vi "Get_DSC_Vals.vi"(8 "Machine":string, 9 "Shared Variable Control":refnum<k21>, 10 "Name":string, 11 "Authorization Header":T1[](array[typedef])) -> ()   [LabVIEW 2016]
uses:
  <vilib>/addons/_JKI.lib/REST Client/classes/REST Client/HTTP Header.ctl
  <vilib>/LVH/i3 JSON/JSON Parsing/Get Object Parameter Files/Get Object Parameter - Object.vi
  <vilib>/LVH/i3 JSON/JSON Parsing/Get Object Parameter Files/Get Object Parameter - String.vi
  <vilib>/addons/_JKI.lib/REST Client/classes/REST Client/REST Client.lvclass
  <vilib>/addons/_JKI.lib/Serialization/JSON/JKI JSON Serialization.lvlib
  <vilib>/LVH/i3 JSON/i3-json.lvlib
panel:
  in  "OK":bool
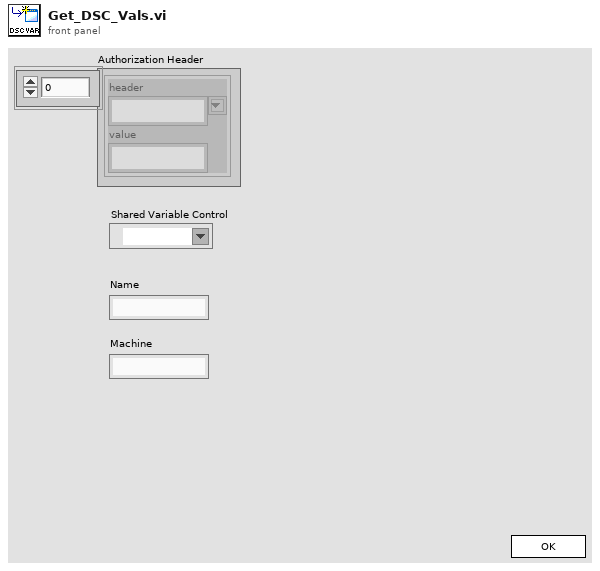
[diagram p1: front panel]
types:
  T1 = typedef "REST Client.lvlib/REST Client.lvclass/HTTP Header.ctl" = cluster{"header":string, "value":string}
  T2 = enum32{"Invalid", "Standard", "Closed", "Hidden", "Minimized", "Maximized"}
  T3 = enum32{"invalid app kind", "Development System", "Run Time System", "Student Edition", "Embedded LabVIEW", "Evaluation", "Custom"}
  T4 = cluster{"Core":cluster{"Current VI Reference":refnum<vi>, "Close Panel on Exit?":bool}, "New Reference":string, "Array of DSC References":cluster{string, string}[], "Authorization Header":T1[], "GID":string, "Name":string, "trimmed string":string, "Section GID":string}
  T5 = cluster{"Current VI Reference":refnum<vi>, "Close Panel on Exit?":bool}
  T6 = cluster{"data":cluster{"id":i32, "gid":string, "name":string, "resource_type":string}[]}
  T7 = cluster{"id":i32, "gid":string, "name":string, "resource_type":string}[]
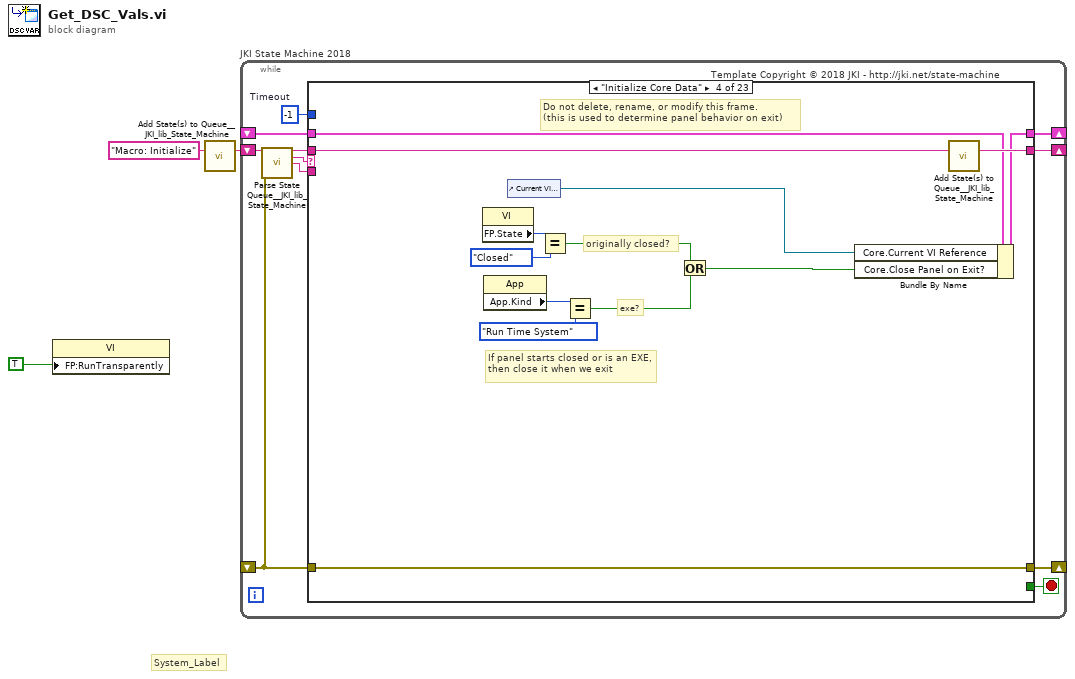
[diagram p0: block diagram]
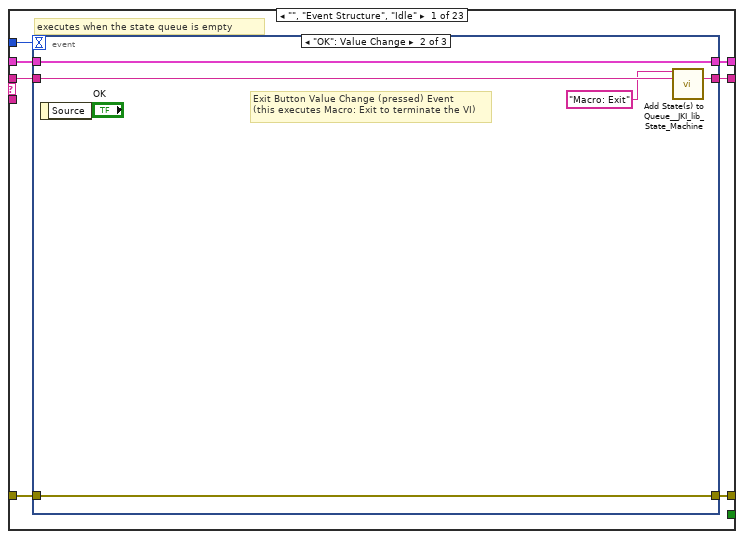
[diagram p2: hidden frame]
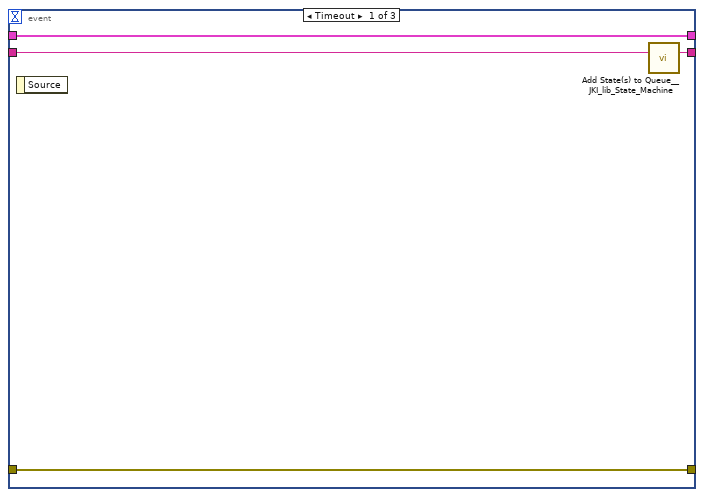
[diagram p3: hidden frame]
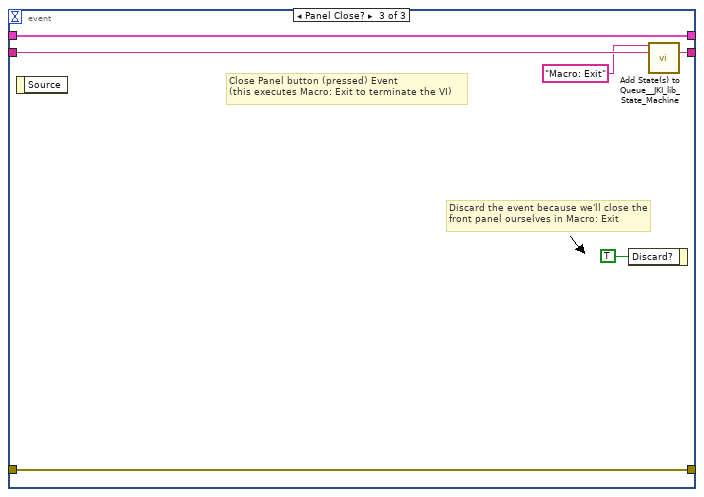
[diagram p4: hidden frame]
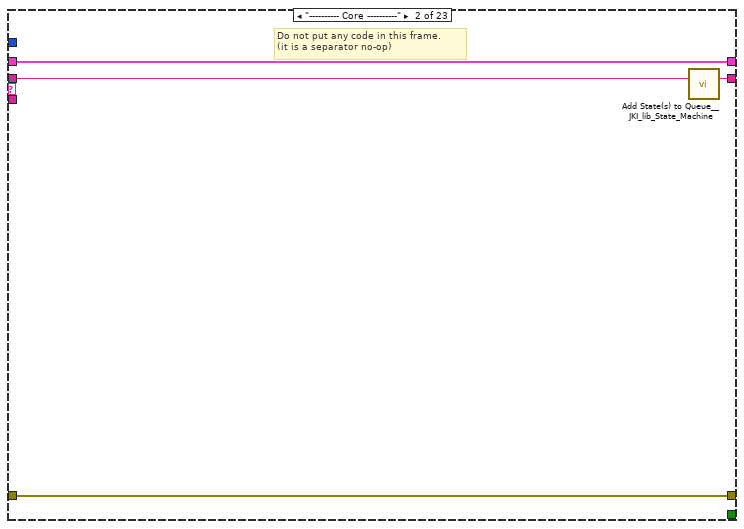
[diagram p5: hidden frame]
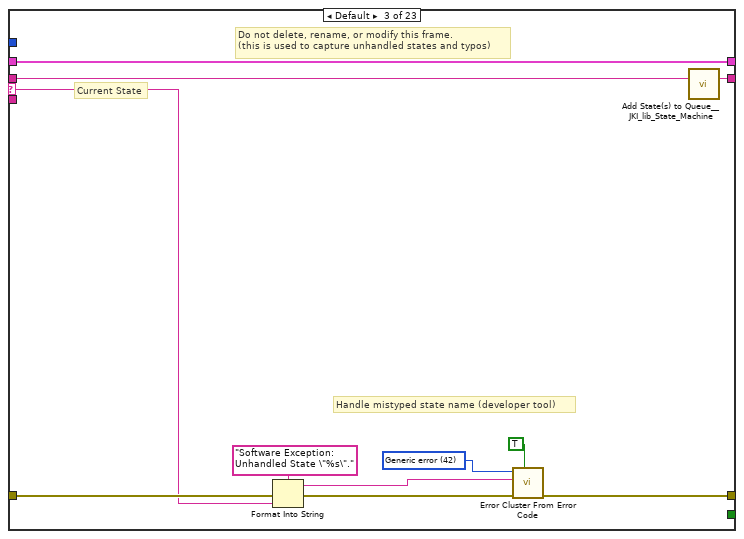
[diagram p6: hidden frame]
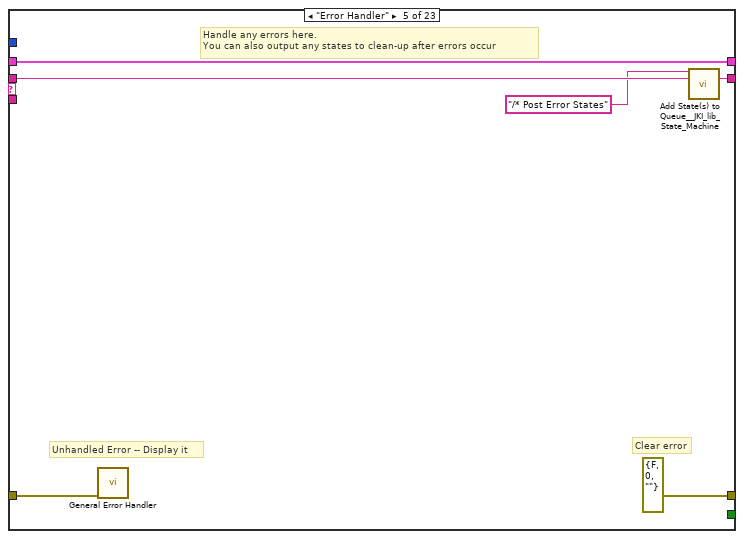
[diagram p7: hidden frame]
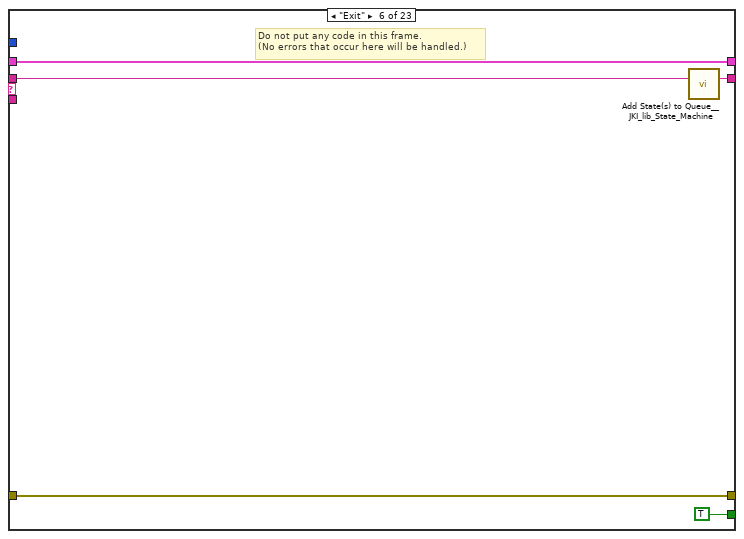
[diagram p8: hidden frame]
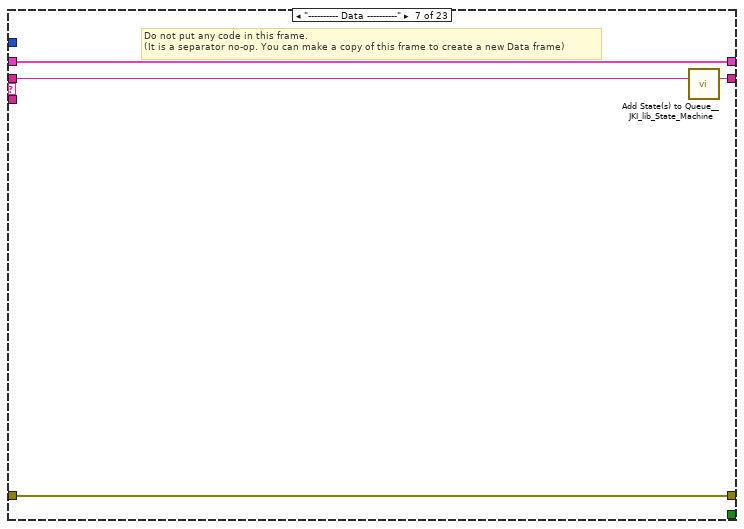
[diagram p9: hidden frame]
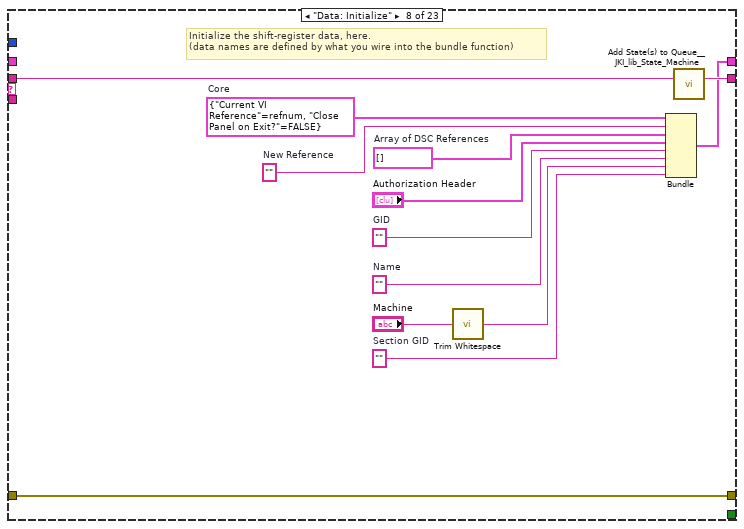
[diagram p10: hidden frame]
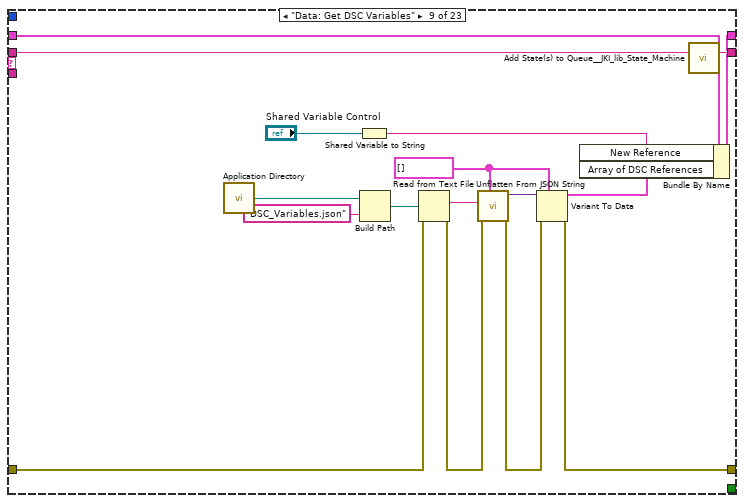
[diagram p11: hidden frame]
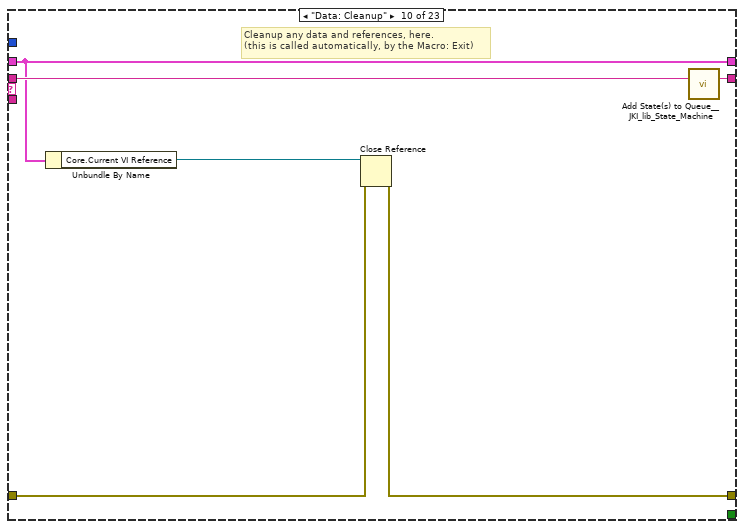
[diagram p12: hidden frame]
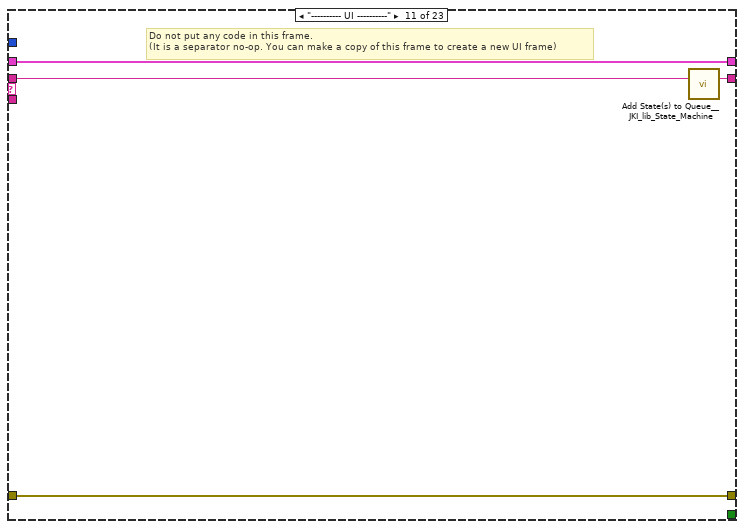
[diagram p13: hidden frame]
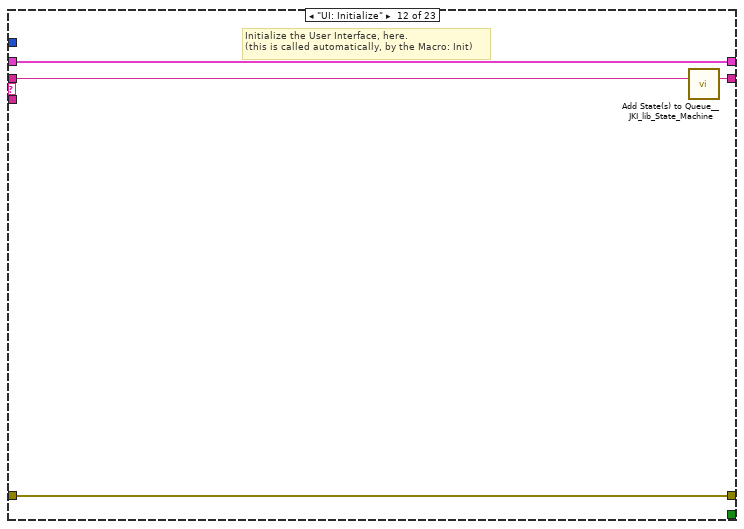
[diagram p14: hidden frame]
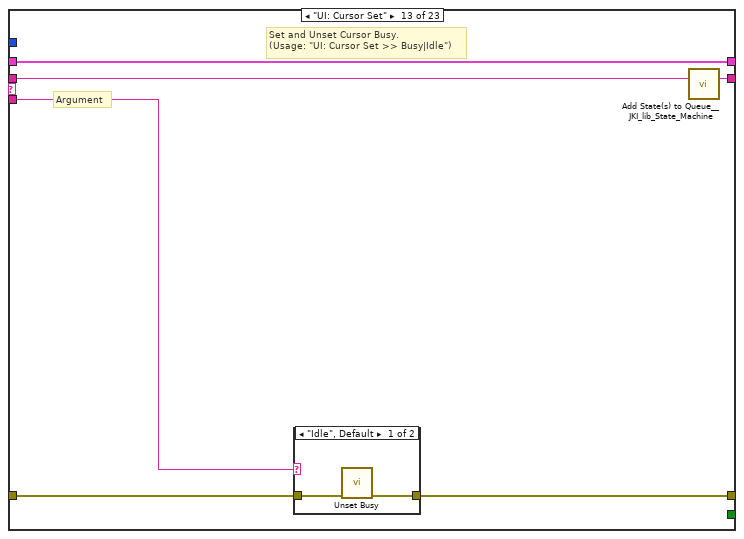
[diagram p15: hidden frame]
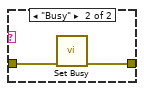
[diagram p16: hidden frame]
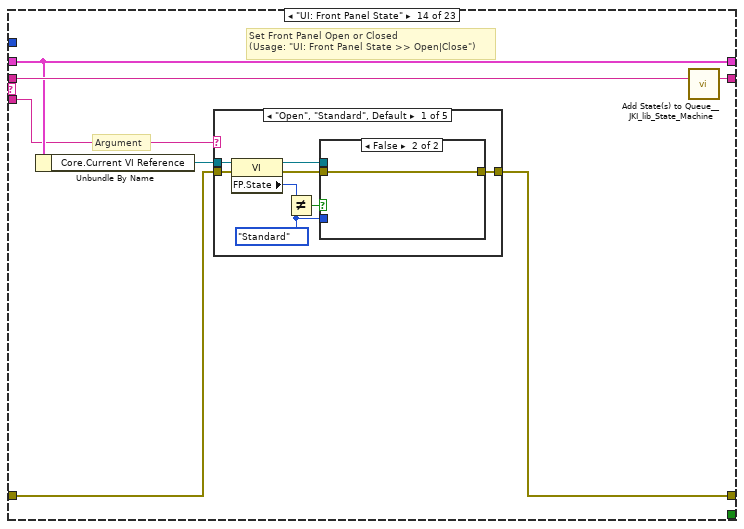
[diagram p17: hidden frame]
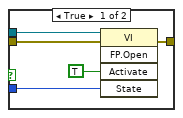
[diagram p18: hidden frame]
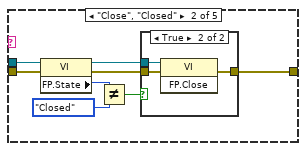
[diagram p19: hidden frame]
diagram:
  # "System_Label"
  n1 = property class="VI"("FP:RunTransparently"=TRUE) -> ()  [unwired: 2 in, 2 out]
  n2 = call <vilib>:"Add State(s) to Queue__JKI_lib_State_Machine.vi"("State(s) in (\"\")"="Macro: Initialize") -> ("States Out"=w3:string)  [unwired: 14 in]
  n3 = while "JKI State Machine 2018" {
    shift-right: [w7] -> _
    shift-left: _ -> [w6]
    shift-right: [w10] -> _
    shift-left: _ -> [w4]
    shift-right: [w9] -> _
    shift-left: w3 -> [w11]
    stop <- w8 stop-if-true
    w5 = -1  # Timeout
    # "Template Copyright © 2018 JKI - http://jki.net/state-machine"
    n4 = call <vilib>:"Parse State Queue__JKI_lib_State_Machine.vi"("State Queue"=w11, "Error In (no error)"=w4) -> ("Remaining States"=w13:string, "Current State"=w14:string, "Arguments"=w12:string)  [unwired: 11 in]
    n5 = case shown="\"Initialize Core Data\"" w14 {
      selector: w14 -> [_ _ w41 _ _ _ _ _ _ _ _ _ _ _ _ _ _ _ _ _ _ _ _]
      tunnel: w13 -> [w21 w40 w45 w64 w70 w75 w79 w92 w109 w115 w119 w123 w129 w140 w209 w214 w224 w228 w238 w270 w308 w334 w364]
      tunnel: w12 -> [_ _ _ _ _ _ _ _ _ _ _ _ w124 w134 _ _ _ _ _ _ _ _ _]
      tunnel: w6 -> [w19 w37 w43 w57 w67 w73 w76 _ w106 w110 w116 w121 w127 w136 w206 w211 w221 w225 w235 w247 w302 w325 w362]
      tunnel: [w18 w38 w47 w61 errorcluster {"status"=FALSE, "code"=0, "source"=""} ("error out") w72 w77 w89 w97 w111 w117 w120 w125 w137 w207 w212 w222 w226 w236 w256 w297 w317 w358] -> w10
      tunnel: w4 -> [w17 w38 w46 w61 w66 w72 w77 w89 w96 w112 w117 w120 w126 w138 w207 w212 w222 w226 w236 w261 w300 w323 w359]
      tunnel: [w20 w39 w44 w63 w69 w74 w78 w91 w108 w114 w118 w122 w128 w139 w208 w213 w223 w227 w237 w269 w307 w333 w363] -> w9
      tunnel: [_ _ _ _ _ TRUE _ _ _ _ _ _ _ _ _ _ _ _ _ _ _ _ _] -> w8
      tunnel: [w16 w37 w43 w62 w67 w73 w76 w90 w105 w110 w116 w121 w127 w136 w206 w211 w221 w225 w235 w246 w301 w324 w362] -> w7
      tunnel: w5 -> [w15 _ _ _ _ _ _ _ _ _ _ _ _ _ _ _ _ _ _ _ _ _ _]
      frame "", "Event Structure", "Idle" {
        # "executes when the state queue is empty"
        n6 = event shown="[1] \"OK\": Value Change" {
          selector: _ -> [_ _ _]
          dyn-events: _ -> [_ _ _]
          timeout: w15 -> [_ _ _]
          tunnel: w21 -> [w25 w30 w36]
          tunnel: [w24 w29 w35] -> w20
          tunnel: w19 -> [w22 w27 w33]
          tunnel: [w23 w28 w34] -> w18
          tunnel: w17 -> [w23 w28 w34]
          tunnel: [w22 w27 w33] -> w16
          event Timeout {
            n7 = event-data() -> ()  [unwired: 1 in, 1 out]
            n8 = call <vilib>:"Add State(s) to Queue__JKI_lib_State_Machine.vi"("State(s) in (\"\")"=w25) -> ("States Out"=w24:string)  [unwired: 14 in]
          }
          event "OK": Value Change {
            # "Exit Button Value Change (pressed) Event\n(this executes Macro: Exit to terminate the VI)"
            n9 = event-data() -> ()  [unwired: 1 in, 1 out]
            n10 = call <vilib>:"Add State(s) to Queue__JKI_lib_State_Machine.vi"("State(s) in Front (\"\")"="Macro: Exit", "State(s) in (\"\")"=w30) -> ("States Out"=w29:string)  [unwired: 13 in]
          }
          event Panel Close? {
            # "Discard the event because we'll close the front panel ourselves in Macro: Exit"
            # "Close Panel button (pressed) Event\n(this executes Macro: Exit to terminate the VI)"
            n11 = event-data() -> ()  [unwired: 1 in, 1 out]
            n12 = event-data("Discard?"=TRUE) -> ()  [unwired: 1 in, 1 out]
            n13 = call <vilib>:"Add State(s) to Queue__JKI_lib_State_Machine.vi"("State(s) in Front (\"\")"="Macro: Exit", "State(s) in (\"\")"=w36) -> ("States Out"=w35:string)  [unwired: 13 in]
          }
        }
      }
      frame "---------- Core ----------" {
        # "Do not put any code in this frame.\n(it is a separator no-op)"
        n14 = call <vilib>:"Add State(s) to Queue__JKI_lib_State_Machine.vi"("State(s) in (\"\")"=w40) -> ("States Out"=w39:string)  [unwired: 14 in]
      }
      frame Default {
        w50 = 42 items=["No error", "Argument error", "Memory is full", "Out of zone", "End of file", "File already open", "Generic file I/O error", "File not found", "File permission error", "Disk is full", "Duplicate path", "Too many files open", "System feature not enabled", "Resource file not found", "Cannot add resource", "Resource not found", "Image not found", "Image memory error", "Pen does not exist", "Config type invalid", "Config token not found", "Config parse error", "Config memory error", "Bad external code format", "Bad external code offset", "External code not present", "Null window", "Destroy window error", "Null menu", "Print aborted", "Bad print record", "Print driver error", "Windows error during printing", "Memory error during printing", "Print dialog error", "Generic print error", "Invalid device refnum", "Device not found", "Device parameter error", "Device unit error", "Cannot open device", "Device call aborted", "Generic error", "Cancelled by user", "Object ID too low", "Object ID too high", "Object not in heap", "Unknown heap", "Unknown object (invalid DefProc)", "Unknown object (DefProc not in table)", "Message out of range", "Invalid (null) method", "Unknown message", "Manager call not supported", "Bad address", "Network operation in progress", "Network operation timed out", "Connection is busy", "Network attribute not supported", "Network error", "Address in use", "System out of memory", "Connection aborted", "Connection refused", "Not connected", "Already connected", "Connection closed", "Initialization error (interapplication manager)", "Bad occurrence", "Wait on unbound occurrence handler", "Occurrence queue overflow", "Datalog type conflict", "Unused", "Unrecognized type (interapplication manager)", "Memory corrupt", "Failed to make temporary DLL", "Old CIN version", "Drag socket not found", "Failed to load drop-object", "Failed to register OLE object", "Failed to release OLE object", "Format specifier type mismatch", "Unknown format specifier", "Too few format specifiers", "Too many format specifiers", "Scan failed", "Newer CIN version", "Error converting to variant", "Runtime menu error", "Password tampered", "Variant attribute not found", "Incompatible variant data type", "Event data is not available", "Event Store is not present", "Occurrence is not found", "Event Queue is not created", "Event info is not available", "Refnum passed is NULL", "Error retrieving Class GUID", "Error retrieving CoClass GUID", "Error retrieving TypeLib GUID.", "Bad built application magic bytes.", "Specific driver is different from the specific driver associated with the Logical Name.", "There is no session opened to the class driver.", "Max Error", "MAX - Error with config objects", "MAX - Error loading configuration", "MAX - Group not supported"]
        # "Current State"
        # "Do not delete, rename, or modify this frame.\n(this is used to capture unhandled states and typos)"
        # "Handle mistyped state name (developer tool)"
        n15 = Format Into String(format string="Software Exception: Unhandled State \"%s\"." ("message"), error in=w46, w41) -> (resulting string=w49:string, error out=w48:errorcluster)  [unwired: 1 in]
        n16 = call <vilib>:"Error Cluster From Error Code.vi"("show call chain? (False)"=TRUE, "error in (no error)"=w48, "error message (\"\")"=w49, "error code (0)"=w50) -> ("error out"=w47:errorcluster)  [unwired: 5 in]
        n17 = call <vilib>:"Add State(s) to Queue__JKI_lib_State_Machine.vi"("State(s) in (\"\")"=w45) -> ("States Out"=w44:string)  [unwired: 14 in]
      }
      frame "Initialize Core Data" {
        # "Do not delete, rename, or modify this frame.\n(this is used to determine panel behavior on exit)"
        # "originally closed?"
        # "exe?"
        # "If panel starts closed or is an EXE, then close it when we exit"
        n18 = property class="VI"() -> ("FP.State"=w54:T2)  [unwired: 2 in, 2 out]
        n19 = property class="App"() -> ("App.Kind"=w60:T3)  [unwired: 2 in, 2 out]
        n20 = control-ref of="Current VI Reference"() -> (w55:refnum<vi>)
        n21 = Equal?(x=w54, y=T2."Closed" ("Front Panel Window:State")) -> (x = y?=w52:bool)
        n22 = Equal?(x=w60, y=T3."Run Time System" ("Application:Kind")) -> (x = y?=w58:bool)
        n23 = Or(x=w52, y=w58) -> (x .or. y?=w56:bool)
        n24 = Bundle By Name(cluster=w57, "Core.Current VI Reference"=w55, "Core.Close Panel on Exit?"=w56) -> (w62:T4)
        n25 = call <vilib>:"Add State(s) to Queue__JKI_lib_State_Machine.vi"("State(s) in (\"\")"=w64) -> ("States Out"=w63:string)  [unwired: 14 in]
      }
      frame "Error Handler" {
        # "Unhandled Error -- Display it"
        # "Handle any errors here.\nYou can also output any states to clean-up after errors occur"
        # "Clear error"
        n26 = call <vilib>:"General Error Handler.vi"("error in (no error)"=w66) -> ()  [unwired: 10 in, 5 out]
        n27 = call <vilib>:"Add State(s) to Queue__JKI_lib_State_Machine.vi"("State(s) in Front (\"\")"="/* Post Error States", "State(s) in (\"\")"=w70) -> ("States Out"=w69:string)  [unwired: 13 in]
      }
      frame "Exit" {
        # "Do not put any code in this frame.\n(No errors that occur here will be handled.)"
        n28 = call <vilib>:"Add State(s) to Queue__JKI_lib_State_Machine.vi"("State(s) in (\"\")"=w75) -> ("States Out"=w74:string)  [unwired: 14 in]
      }
      frame "---------- Data ----------" {
        # "Do not put any code in this frame.\n(It is a separator no-op. You can make a copy of this frame to create a new Data frame)"
        n29 = call <vilib>:"Add State(s) to Queue__JKI_lib_State_Machine.vi"("State(s) in (\"\")"=w79) -> ("States Out"=w78:string)  [unwired: 14 in]
      }
      frame "Data: Initialize" {
        w80 = ""  # Section GID
        w83 = ""  # Name
        w84 = ""  # GID
        w86 = ""  # New Reference
        w87 = cluster{string, string}[] []  # Array of DSC References
        w88 = T5 {"Current VI Reference"=refnum, "Close Panel on Exit?"=FALSE}  # Core
        # "Initialize the shift-register data, here.\n(data names are defined by what you wire into the bundle function)"
        n30 = call <vilib>:"Trim Whitespace.vi"("string"="Machine") -> ("trimmed string"=w81:string)  [unwired: 1 in]
        n31 = Bundle("Core"=w88, "New Reference"=w86, "Array of DSC References"=w87, "Authorization Header"="Authorization Header", "GID"=w84, "Name"=w83, "trimmed string"=w81, "Section GID"=w80) -> (w90:T4)  [unwired: 1 in]
        n32 = call <vilib>:"Add State(s) to Queue__JKI_lib_State_Machine.vi"("State(s) in (\"\")"=w92) -> ("States Out"=w91:string)  [unwired: 14 in]
      }
      frame "Data: Get DSC Variables" {
        w93 = cluster{string, string}[] []
        n33 = call <vilib>:"Application Directory.vi"() -> ("Application Directory"=w102:path)
        n34 = Shared Variable to String(1:"Shared Variable Control") -> (0:w104:string)
        n35 = Build Path(base path=w102, name or relative path="DSC_Variables.json") -> (appended path=w101:path)
        n36 = Read from Text File(file (use dialog)=w101, error in=w96) -> (text=w98:string, error out=w95:errorcluster)  [unwired: 2 in, 2 out]
        n37 = call <vilib>:"Unflatten From JSON String.vi"("Type and Defaults"=w93, "error in (no error)"=w95, "JSON String"=w98) -> ("error out"=w94:errorcluster, "Variant"=w100:variant)  [unwired: 7 in]
        n38 = Variant To Data(error in=w94, type=w93, Variant=w100) -> (data=w99:cluster{string, string}[], error out=w97:errorcluster)
        n39 = Bundle By Name(cluster=w106, "New Reference"=w104, "Array of DSC References"=w99) -> (w105:T4)
        n40 = call <vilib>:"Add State(s) to Queue__JKI_lib_State_Machine.vi"("State(s) in (\"\")"=w109) -> ("States Out"=w108:string)  [unwired: 14 in]
      }
      frame "Data: Cleanup" {
        # "Cleanup any data and references, here.\n(this is called automatically, by the Macro: Exit)"
        n41 = Unbundle By Name(w110) -> ("Core.Current VI Reference"=w113:refnum<vi>)
        n42 = Close Reference(reference=w113, error in (no error)=w112) -> (error out=w111:errorcluster)
        n43 = call <vilib>:"Add State(s) to Queue__JKI_lib_State_Machine.vi"("State(s) in (\"\")"=w115) -> ("States Out"=w114:string)  [unwired: 14 in]
      }
      frame "---------- UI ----------" {
        # "Do not put any code in this frame.\n(It is a separator no-op. You can make a copy of this frame to create a new UI frame)"
        n44 = call <vilib>:"Add State(s) to Queue__JKI_lib_State_Machine.vi"("State(s) in (\"\")"=w119) -> ("States Out"=w118:string)  [unwired: 14 in]
      }
      frame "UI: Initialize" {
        # "Initialize the User Interface, here.\n(this is called automatically, by the Macro: Init)"
        n45 = call <vilib>:"Add State(s) to Queue__JKI_lib_State_Machine.vi"("State(s) in (\"\")"=w123) -> ("States Out"=w122:string)  [unwired: 14 in]
      }
      frame "UI: Cursor Set" {
        # "Argument"
        # "Set and Unset Cursor Busy.\n(Usage: \"UI: Cursor Set >> Busy|Idle\")"
        n46 = case shown="\"Idle\", Default" w124 {
          tunnel: w126 -> [w131 w133]
          tunnel: [w130 w132] -> w125
          frame "Idle", Default {
            n47 = call <vilib>:"Unset Busy.vi"("error in (no error)"=w131) -> ("error out"=w130:errorcluster)  [unwired: 10 in]
          }
          frame "Busy" {
            n48 = call <vilib>:"Set Busy.vi"("error in (no error)"=w133) -> ("error out"=w132:errorcluster)  [unwired: 9 in, 1 out]
          }
        }
        n49 = call <vilib>:"Add State(s) to Queue__JKI_lib_State_Machine.vi"("State(s) in (\"\")"=w129) -> ("States Out"=w128:string)  [unwired: 14 in]
      }
      frame "UI: Front Panel State" {
        # "Argument"
        # "Set Front Panel Open or Closed\n(Usage: \"UI: Front Panel State >> Open|Close\")"
        n50 = Unbundle By Name(w136) -> ("Core.Current VI Reference"=w135:refnum<vi>)
        n51 = case shown="\"Open\", \"Standard\", Default" w134 {
          tunnel: w138 -> [w146 w161 w172 w185 w198]
          tunnel: [w148 w162 w174 w187 w200] -> w137
          tunnel: w135 -> [w147 w159 w173 w186 w199]
          frame "Open", "Standard", Default {
            w141 = T2."Standard" ("State")
            n52 = property class="VI"(reference=w147, error in=w146) -> (reference out=w144:refnum<vi>, error out=w145:errorcluster, "FP.State"=w143:T2)
            n53 = Not Equal?(x=w143, y=w141) -> (x != y?=w142:bool)
            n54 = case shown="False" w142 {
              tunnel: [w152 w154] -> w148
              tunnel: w145 -> [w151 w154]
              tunnel: w144 -> [w150 _]
              tunnel: w141 -> [w149 _]
              frame True {
                n55 = invoke class="VI" method="FP.Open"(reference=w150, error in=w151, "Activate"=TRUE, "State"=w149) -> (error out=w152:errorcluster)  [unwired: 1 in, 4 out]
              }
              frame False {
              }
            }
          }
          frame "Close", "Closed" {
            n56 = property class="VI"(reference=w159, error in=w161) -> (reference out=w158:refnum<vi>, error out=w160:errorcluster, "FP.State"=w156:T2)
            n57 = Not Equal?(x=w156, y=T2."Closed" ("Front Panel Window:State")) -> (x != y?=w155:bool)
            n58 = case shown="True" w155 {
              tunnel: [w163 w166] -> w162
              tunnel: w160 -> [w163 w165]
              tunnel: w158 -> [_ w164]
              frame False {
              }
              frame True {
                n59 = invoke class="VI" method="FP.Close"(reference=w164, error in=w165) -> (error out=w166:errorcluster)  [unwired: 1 in, 2 out]
              }
            }
          }
          frame "Hidden", "Hide" {
            w167 = T2."Hidden" ("State")
            n60 = property class="VI"(reference=w173, error in=w172) -> (reference out=w170:refnum<vi>, error out=w171:errorcluster, "FP.State"=w169:T2)
            n61 = Not Equal?(x=w169, y=w167) -> (x != y?=w168:bool)
            n62 = case shown="True" w168 {
              tunnel: [w178 w179] -> w174
              tunnel: w171 -> [w177 w179]
              tunnel: w170 -> [w176 _]
              tunnel: w167 -> [w175 _]
              frame True {
                n63 = invoke class="VI" method="FP.Open"(reference=w176, error in=w177, "State"=w175) -> (error out=w178:errorcluster)  [unwired: 2 in, 4 out]
              }
              frame False {
              }
            }
          }
          frame "Minimize", "Minimized" {
            w180 = T2."Minimized" ("State")
            n64 = property class="VI"(reference=w186, error in=w185) -> (reference out=w183:refnum<vi>, error out=w184:errorcluster, "FP.State"=w182:T2)
            n65 = Not Equal?(x=w182, y=w180) -> (x != y?=w181:bool)
            n66 = case shown="True" w181 {
              tunnel: [w191 w192] -> w187
              tunnel: w184 -> [w190 w192]
              tunnel: w183 -> [w189 _]
              tunnel: w180 -> [w188 _]
              frame True {
                n67 = invoke class="VI" method="FP.Open"(reference=w189, error in=w190, "State"=w188) -> (error out=w191:errorcluster)  [unwired: 2 in, 4 out]
              }
              frame False {
              }
            }
          }
          frame "Maximize", "Maximized" {
            w193 = T2."Maximized" ("State")
            n68 = property class="VI"(reference=w199, error in=w198) -> (reference out=w196:refnum<vi>, error out=w197:errorcluster, "FP.State"=w195:T2)
            n69 = Not Equal?(x=w195, y=w193) -> (x != y?=w194:bool)
            n70 = case shown="True" w194 {
              tunnel: [w204 w205] -> w200
              tunnel: w197 -> [w203 w205]
              tunnel: w196 -> [w202 _]
              tunnel: w193 -> [w201 _]
              frame True {
                n71 = invoke class="VI" method="FP.Open"(reference=w202, error in=w203, "State"=w201) -> (error out=w204:errorcluster)  [unwired: 2 in, 4 out]
              }
              frame False {
              }
            }
          }
        }
        n72 = call <vilib>:"Add State(s) to Queue__JKI_lib_State_Machine.vi"("State(s) in (\"\")"=w140) -> ("States Out"=w139:string)  [unwired: 14 in]
      }
      frame "---------- Macro ----------" {
        # "Do not put any code in this frame.\n(It is a separator no-op. You can make a copy of this frame to create a new Macro frame)"
        n73 = call <vilib>:"Add State(s) to Queue__JKI_lib_State_Machine.vi"("State(s) in (\"\")"=w209) -> ("States Out"=w208:string)  [unwired: 14 in]
      }
      frame "Macro: Initialize" {
        # "Initialization Macro\n(This is called once, when the VI starts)"
        n74 = call <vilib>:"Add State(s) to Queue__JKI_lib_State_Machine.vi"("State(s) in Front (\"\")"="Data: Initialize\nInitialize Core Data\nUI: Initialize\nUI: Front Panel State >> Open\nData: Get DSC Variables\nOperations: Check List", "State(s) in (\"\")"=w214) -> ("States Out"=w213:string)  [unwired: 13 in]
      }
      frame "Macro: Exit" {
        # "Exit Macro\n(This is called once, when the VI exits)"
        n75 = Unbundle By Name(w221) -> ("Core.Close Panel on Exit?"=w220:bool)
        n76 = Select(t="UI: Front Panel State >> Close", s=w220, f="") -> (s? t:f=w217:string)
        n77 = call <vilib>:"Add State(s) to Queue__JKI_lib_State_Machine.vi"("State(s) in (\"\")"=w217, "State(s) at Back (\"\")"="Data: Cleanup\nExit") -> ("States Out"=w215:string)  [unwired: 13 in]
        n78 = call <vilib>:"Add State(s) to Queue__JKI_lib_State_Machine.vi"("State(s) in Front (\"\")"=w215, "State(s) in (\"\")"=w224) -> ("States Out"=w223:string)  [unwired: 13 in]
      }
      frame "---------- Operations ----------" {
        # "Template Separator\n(You can make a copy of, or modify, this frame)"
        n79 = call <vilib>:"Add State(s) to Queue__JKI_lib_State_Machine.vi"("State(s) in (\"\")"=w228) -> ("States Out"=w227:string)  [unwired: 14 in]
      }
      frame "Operations: Check List" {
        # "Your code here.\n(You can make a copy of, or modify, this frame)"
        n80 = Unbundle By Name(w235) -> ("Array of DSC References"=w234:cluster{string, string}[], "New Reference"=w233:string)
        n81 = for {
          tunnel: w234 -> [w243] mode=indexing
          tunnel: w233 -> [w242]
          tunnel: [w241] -> w231 mode=indexing
          stop <- w241 stop-if-true
          n82 = Unbundle(w243) -> (w244:string)  [unwired: 1 out]
          n83 = Equal?(x=w244, y=w242) -> (x = y?=w241:bool)
        }
        n84 = Search 1D Array(1D array=w231, element=TRUE) -> (index of element=w229:i32)  [unwired: 1 in]
        n85 = case shown="-1" w229 {
          tunnel: ["Macro: Exit" "Operations: Check Section\nOperations: Make Asana Task\nOperations: Add to List"] -> w232
          frame 0, Default {
            n86 = call "Display Message to User"() -> ()  [unwired: 10 in, 2 out]
          }
          frame -1 {
          }
        }
        n87 = call <vilib>:"Add State(s) to Queue__JKI_lib_State_Machine.vi"("State(s) in Front (\"\")"=w232, "State(s) in (\"\")"=w238) -> ("States Out"=w237:string)  [unwired: 13 in]
      }
      frame "Operations: Check Section" {
        w263 = T6 {"data"=[]}
        # "Your code here.\n(You can make a copy of, or modify, this frame)"
        n88 = Unbundle By Name(w247) -> ("Authorization Header"=w255:T1[], "trimmed string"=w250:string)
        n89 = call <vilib>:"Create REST Client.vi"("error in (no error)"=w261, "Base URL"="https://app.asana.com/api/1.0") -> ("error out"=w260:errorcluster, "REST Client out"=w268:refnum<class "REST Client.lvclass">)  [unwired: 8 in]
        n90 = call-dynamic "HTTP GET.vi"("request specific headers"=w255, "error in (no error)"=w260, "Path"="/projects/1122243734894450/sections", "REST Client in"=w268) -> ("error out"=w259:errorcluster, "Response body"=w262:string, "REST Client out"=w267:refnum<class "REST Client.lvclass">)  [unwired: 2 in, 3 out]
        n91 = call-dynamic "Destroy REST Client.vi"("error in (no error)"=w259, "REST Client in"=w267) -> ("error out"=w258:errorcluster)  [unwired: 9 in]
        n92 = call <vilib>:"Unflatten From JSON String.vi"("Type and Defaults"=w263, "error in (no error)"=w258, "JSON String"=w262) -> ("error out"=w257:errorcluster, "Variant"=w264:variant)  [unwired: 7 in]
        n93 = Variant To Data(error in=w257, type=w263, Variant=w264) -> (data=w254:T6, error out=w256:errorcluster)
        n94 = Unbundle(w254) -> ("data"=w253:T7)
        n95 = for {
          tunnel: w253 -> [w279] mode=indexing
          tunnel: [w278] -> w252 mode=indexing
          tunnel: [w277] -> w248 mode=indexing
          n96 = Unbundle By Name(w279) -> ("gid"=w277:string, "name"=w278:string)
        }
        n97 = Search 1D Array(1D array=w252, element=w250) -> (index of element=w251:i32)  [unwired: 1 in]
        n98 = case shown="-1" w251 {
          selector: w251 -> [w273 _]
          tunnel: ["" "Operations: Make Section"] -> w249
          tunnel: w248 -> [w274 _]
          tunnel: [w272 ""] -> w245
          frame 0, Default {
            n99 = Index Array(array=w274, index=w273) -> (element=w272:string)
          }
          frame -1 {
          }
        }
        n100 = Bundle By Name(cluster=w247, "Section GID"=w245) -> (w246:T4)
        n101 = call <vilib>:"Add State(s) to Queue__JKI_lib_State_Machine.vi"("State(s) in Front (\"\")"=w249, "State(s) in (\"\")"=w270) -> ("States Out"=w269:string)  [unwired: 13 in]
      }
      frame "Operations: Make Asana Task" {
        n102 = Unbundle By Name(w302) -> ("Section GID"=w292:string, "Authorization Header"=w296:T1[])
        n103 = Concatenate Strings("{\"data\": { \"name\":  \"" ("Request body"), "Name", " = \", \"projects\": \"1122243734894450\", \"memberships\": [{\"project\": \"1122243734894450\", \"section\": \"", w292, "\"}]}}" ("string")) -> (w295:string)
        n104 = call <vilib>:"Create REST Client.vi"("error in (no error)"=w300, "Base URL"="https://app.asana.com/api/1.0") -> ("error out"=w299:errorcluster, "REST Client out"=w306:refnum<class "REST Client.lvclass">)  [unwired: 8 in]
        n105 = call-dynamic "HTTP POST.vi"("request specific headers"=w296, "error in (no error)"=w299, "Request body"=w295, "Path"="/tasks", "REST Client in"=w306) -> ("error out"=w281:errorcluster, "Response body"=w285:string, "REST Client out"=w293:refnum<class "REST Client.lvclass">)  [unwired: 1 in, 3 out]
        n106 = call <vilib>:"Parse JSON.vi"("error in (no error)"=w281, "JSON String"=w285) -> ("error out"=w282:errorcluster, "JSON Tree"=w289:variant)  [unwired: 6 in, 2 out]
        n107 = call-poly <vilib>:"Get Object Parameter.vi"("error in (no error)"=w282, "Parameter Name"="data", "JSON Tree In (JSON Object)"=w289) -> ("error out"=w283:errorcluster, "JSON Object"=w288:variant)  [unwired: 5 in, 2 out]
        n108 = call-poly <vilib>:"Get Object Parameter.vi"("error in (no error)"=w283, "Parameter Name"="gid", "JSON Tree In (JSON Object)"=w288) -> ("error out"=w284:errorcluster, "String Value"=w280:string)  [unwired: 5 in, 2 out]
        n109 = Bundle By Name(cluster=w302, "GID"=w280, "Name"="Name") -> (w301:T4)
        n110 = call-dynamic "Destroy REST Client.vi"("error in (no error)"=w284, "REST Client in"=w293) -> ("error out"=w297:errorcluster)  [unwired: 9 in]
        n111 = call <vilib>:"Add State(s) to Queue__JKI_lib_State_Machine.vi"("State(s) in (\"\")"=w308, "State(s) at Back (\"\")"="Macro: Exit" ("State(s) in Front (\"\")")) -> ("States Out"=w307:string)  [unwired: 13 in]
      }
      frame "Operations: Make Section" {
        n112 = Unbundle By Name(w325) -> ("trimmed string"=w319:string, "Authorization Header"=w330:T1[])
        n113 = Concatenate Strings("{\"data\": {\"name\":  \"" ("Request body"), w319, "\"}}") -> (w326:string)
        n114 = call <vilib>:"Create REST Client.vi"("error in (no error)"=w323, "Base URL"="https://app.asana.com/api/1.0") -> ("error out"=w321:errorcluster, "REST Client out"=w332:refnum<class "REST Client.lvclass">)  [unwired: 8 in]
        n115 = call-dynamic "HTTP POST.vi"("request specific headers"=w330, "error in (no error)"=w321, "Request body"=w326, "Path"="/projects/1122243734894450/sections", "REST Client in"=w332) -> ("error out"=w322:errorcluster, "Response body"=w314:string, "REST Client out"=w331:refnum<class "REST Client.lvclass">)  [unwired: 1 in, 3 out]
        n116 = call-dynamic "Destroy REST Client.vi"("error in (no error)"=w322, "REST Client in"=w331) -> ("error out"=w318:errorcluster)  [unwired: 9 in]
        n117 = call <vilib>:"Parse JSON.vi"("error in (no error)"=w318, "JSON String"=w314) -> ("error out"=w315:errorcluster, "JSON Tree"=w313:variant)  [unwired: 6 in, 2 out]
        n118 = call-poly <vilib>:"Get Object Parameter.vi"("error in (no error)"=w315, "Parameter Name"="data", "JSON Tree In (JSON Object)"=w313) -> ("error out"=w316:errorcluster, "JSON Object"=w312:variant)  [unwired: 5 in, 2 out]
        n119 = call-poly <vilib>:"Get Object Parameter.vi"("error in (no error)"=w316, "Parameter Name"="gid", "JSON Tree In (JSON Object)"=w312) -> ("error out"=w317:errorcluster, "String Value"=w309:string)  [unwired: 5 in, 2 out]
        n120 = Bundle By Name(cluster=w325, "Section GID"=w309) -> (w324:T4)
        n121 = call <vilib>:"Add State(s) to Queue__JKI_lib_State_Machine.vi"("State(s) in (\"\")"=w334) -> ("States Out"=w333:string)  [unwired: 14 in]
      }
      frame "Operations: Add to List" {
        w339 = cluster{string, string}[] []
        # "Your code here.\n(You can make a copy of, or modify, this frame)"
        n122 = Unbundle By Name(w362) -> ("Name"=w337:string, "New Reference"=w348:string, "GID"=w347:string)
        n123 = call <vilib>:"Application Directory.vi"() -> ("Application Directory"=w357:path)
        n124 = Build Path(base path=w357, name or relative path="DSC_Variables.json") -> (appended path=w338:path)
        n125 = Read from Text File(file (use dialog)=w338, error in=w359) -> (text=w356:string, error out=w355:errorcluster)  [unwired: 2 in, 2 out]
        n126 = Bundle("New Reference"=w348, "GID"=w347) -> (w360:cluster{"New Reference":string, "GID":string})  [unwired: 1 in]
        n127 = call <vilib>:"Application Directory.vi"() -> ("Application Directory"=w346:path)
        n128 = call <vilib>:"Unflatten From JSON String.vi"("Type and Defaults"=w339, "error in (no error)"=w355, "JSON String"=w356) -> ("error out"=w350:errorcluster, "Variant"=w354:variant)  [unwired: 7 in]
        n129 = Build Path(base path=w346, name or relative path="Task_Name_Search.txt") -> (appended path=w340:path)
        n130 = Variant To Data(error in=w350, type=w339, Variant=w354) -> (data=w335:cluster{string, string}[], error out=w349:errorcluster)
        n131 = call <vilib>:"Trim Whitespace.vi"("string"=w337) -> ("trimmed string"=w336:string)  [unwired: 1 in]
        n132 = Read from Text File(file (use dialog)=w340) -> (text=w344:string)  [unwired: 3 in, 3 out]
        n133 = Insert Into Array(array=w335, new element=w360) -> (w353:cluster{string, string}[])  [unwired: 1 in]
        n134 = Concatenate Strings(w344, "|" ("string"), w336, " = " ("string")) -> (w341:string)
        n135 = call <vilib>:"Flatten To JSON String.vi"("error in (no error)"=w349, "Variant"=w353) -> ("error out"=w352:errorcluster, "JSON String"=w351:string)  [unwired: 8 in]
        n136 = Write to Text File(file (use dialog)=w340, text=w341) -> ()  [unwired: 2 in, 3 out]
        n137 = Write to Text File(file (use dialog)=w338, text=w351, error in=w352) -> (error out=w358:errorcluster)  [unwired: 1 in, 2 out]
        n138 = call <vilib>:"Add State(s) to Queue__JKI_lib_State_Machine.vi"("State(s) in (\"\")"=w364) -> ("States Out"=w363:string)  [unwired: 14 in]
      }
    }
  }
